vi "Init.vi"(8 "error in (no error)":errorcluster, 11 "reference in":refnum<class "Switch_Manager.lvclass">) -> (0 "error out":errorcluster, 3 "reference out":refnum<class "Switch_Manager.lvclass">)   [LabVIEW 2022 SP3, in "Switch_Manager.lvlib" / "Switch_Manager.lvclass"]
uses:
  Switch_Manager.lvclass
  Components/SwitchBase.lvlibp/SwitchBase.lvclass
  protected/SwitchMap.ctl
  <userlib>/_OpenG.lib/array/array.llb/Search 1D Array (String)__ogtk.vi
  <userlib>/_OpenG.lib/array/array.llb/Delete Elements from 1D Array (String)__ogtk.vi
  <userlib>/_OpenG.lib/array/array.llb/Remove Duplicates from 1D Array (String)__ogtk.vi
  <userlib>/_OpenG.lib/array/array.llb/Delete Elements from 1D Array (Boolean)__ogtk.vi
  Components/ViPER.lvlibp/ViPER.lvclass
  C:/Projects/Medulla/ViPER/Examples/Flux_Capacitor_Tester/Components/ViPER.lvlibp/ViPER.lvclass
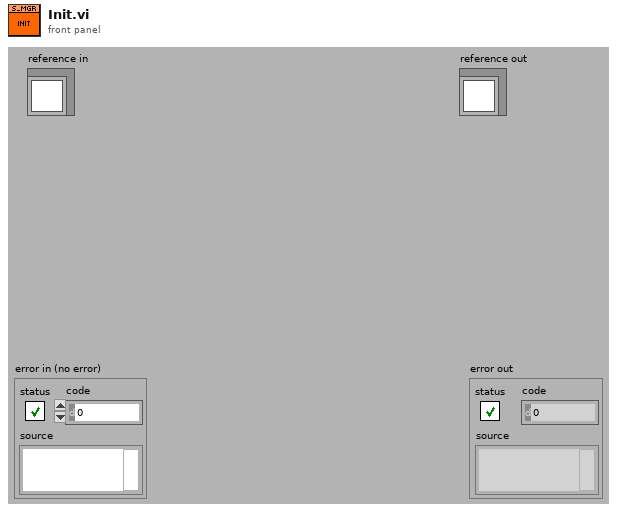
[diagram p1: front panel]
types:
  T1 = typedef "Switch_Manager.lvlib/Switch_Manager.lvclass/SwitchMap.ctl" = cluster{"Name":string, "Description":string, "Group":string, "IsGroup":bool, "Switches":string[]}
  T2 = cluster{"Ancestor":string, "Objects":refnum<class "ViPER.lvclass">[], "Object_Names":string[], "Owned":bool[]}[]
  T3 = cluster{"Ancestor":string, "Objects":refnum<class "ViPER.lvclass">[], "Object_Names":string[], "Owned":bool[]}
  T4 = cluster{"Name":string, "Description":string, "Group":string, "IsGroup":bool}[]
  T5 = typedef "Switch_Manager.lvlib/Switch_Manager.lvclass/ObjectAttributes.ctl" = cluster{"Config":T6, "State":bool[], "Switches":refnum<class "SwitchBase.lvclass">[], "SwitchName":string[], "SwitchMap":T1[], "UpdateEvent":refnum<user-event>, "ParentEvent":refnum<user-event>, "Tree":bool[]}
  T6 = typedef "Switch_Manager.lvlib/Switch_Manager.lvclass/Config.ctl" = cluster{"default":string}
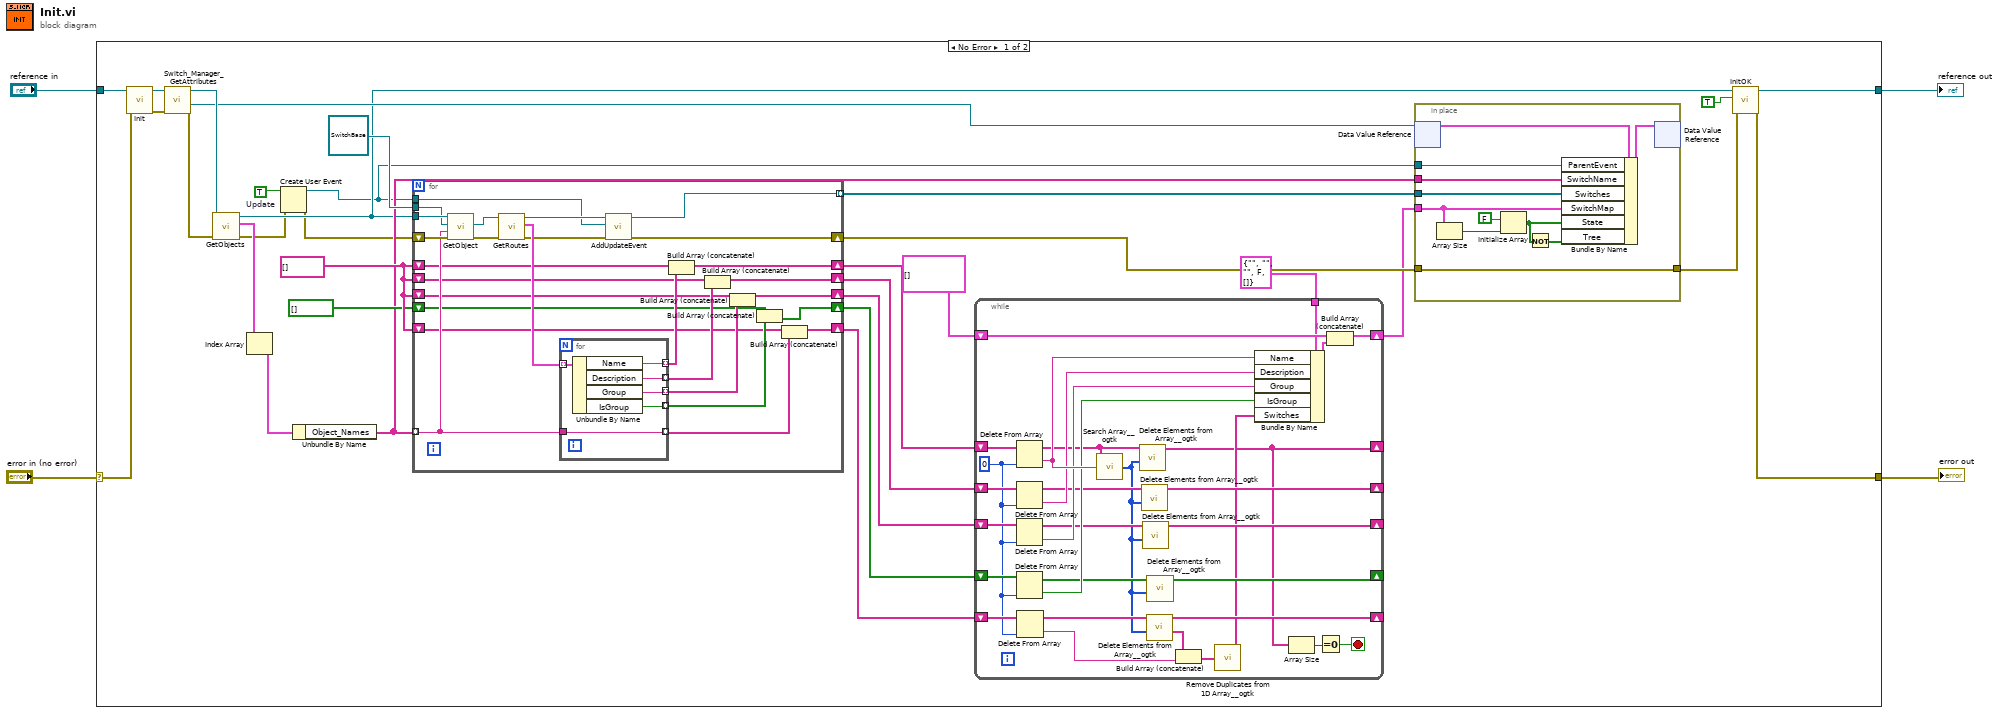
[diagram p0: block diagram]
diagram:
  n1 = case shown="No Error" "error in (no error)" {
    selector: "error in (no error)" -> [w35 w113]
    tunnel: [w30 w113] -> w3
    tunnel: [w32 w112] -> w1
    tunnel: "reference in" -> [w36 w112]
    frame No Error {
      w6 = TRUE  # Update
      w21 = string[] []
      n2 = call-parent "Init.vi"("error in (no error)"=w35, "reference in"=w36) -> ("error out"=w33:errorcluster, "reference out"=w34:refnum<class "Switch_Manager.lvclass">)  [unwired: 8 in]
      n3 = call "Switch_Manager_GetAttributes.vi"("error in (no error)"=w33, "reference in"=w34) -> ("error out"=w29:errorcluster, "DataRef"=w24:refnum<data-value>, "reference out"=w28:refnum<class "Switch_Manager.lvclass">)  [unwired: 6 in, 1 out]
      n4 = call "GetObjects.vi"("error in (no error)"=w29, "reference in"=w28) -> ("error out"=w8:errorcluster, "Ancestors"=w26:T2, "reference out"=w10:refnum<class "Switch_Manager.lvclass">)  [unwired: 7 in]
      n5 = Index Array(array=w26) -> (element=w25:T3)  [unwired: 1 in]
      n6 = Create User Event(user event datatype=w6, error in=w8) -> (user event=w5:refnum<user-event>, error out=w7:errorcluster)
      n7 = Unbundle By Name(w25) -> ("Object_Names"=w12:string[])
      n8 = for {
        tunnel: w10 -> [w94]
        tunnel: refnum<class "SwitchBase.lvclass"> refnum ("SwitchBase.lvlibp:reference") -> [w92]
        tunnel: w12 -> [w88] mode=indexing
        shift-right: [w71] -> w23
        shift-left: w7 -> [w93]
        tunnel: [w69] -> w22 mode=indexing
        shift-right: [w85] -> w19
        shift-left: w21 -> [w87]
        shift-right: [w82] -> w16
        shift-left: w21 -> [w84]
        shift-right: [w79] -> w15
        shift-left: w21 -> [w81]
        shift-right: [w76] -> w14
        shift-left: bool[] [] -> [w78]
        shift-right: [w73] -> w13
        shift-left: w21 -> [w75]
        tunnel: w5 -> [w68]
        n9 = call "GetObject.vi"("error in (no error)"=w93, "Object Name"=w88, "Class type"=w92, "reference in"=w94) -> ("error out"=w91:errorcluster, "Object out"=w90:refnum<class "SwitchBase.lvclass">)  [unwired: 5 in, 1 out]
        n10 = call-dynamic "GetRoutes.vi"("error in (no error)"=w91, "reference in"=w90) -> ("error out"=w72:errorcluster, "Routes"=w89:T4, "reference in"=w70:refnum<class "SwitchBase.lvclass">)  [unwired: 7 in]
        n11 = for {
          tunnel: w89 -> [w100] mode=indexing
          tunnel: w88 -> [w95]
          tunnel: [w99] -> w86 mode=indexing
          tunnel: [w98] -> w83 mode=indexing
          tunnel: [w97] -> w80 mode=indexing
          tunnel: [w96] -> w77 mode=indexing
          tunnel: [w95] -> w74 mode=indexing
          n12 = Unbundle By Name(w100) -> ("Name"=w99:string, "Description"=w98:string, "Group"=w97:string, "IsGroup"=w96:bool)
        }
        n13 = call-dynamic "AddUpdateEvent.vi"("error in (no error)"=w72, "UpdateEvent"=w68, "reference in"=w70) -> ("error out"=w71:errorcluster, "reference in"=w69:refnum<class "SwitchBase.lvclass">)  [unwired: 7 in]
        n14 = Build Array (concatenate)(w87, w86) -> (w85:string[])
        n15 = Build Array (concatenate)(w84, w83) -> (w82:string[])
        n16 = Build Array (concatenate)(w81, w80) -> (w79:string[])
        n17 = Build Array (concatenate)(w78, w77) -> (w76:bool[])
        n18 = Build Array (concatenate)(w75, w74) -> (w73:string[])
      }
      n19 = while {
        shift-right: [w41] -> _
        shift-left: w19 -> [w67]
        shift-right: [w65] -> w11
        shift-left: T1[] [] -> [w66]
        tunnel: T1 {"Name"="", "Description"="", "Group"="", "IsGroup"=FALSE, "Switches"=[]} -> [w64]
        shift-right: [w52] -> _
        shift-left: w16 -> [w62]
        shift-right: [w51] -> _
        shift-left: w15 -> [w60]
        shift-right: [w49] -> _
        shift-left: w14 -> [w59]
        shift-right: [w46] -> _
        shift-left: w13 -> [w55]
        stop <- w39 stop-if-true
        w37 = 0 ("index")
        n20 = Delete From Array(array=w67, index=w37) -> (deleted portion=w63:string, array with subset deleted=w56:string[])  [unwired: 1 in]
        n21 = Delete From Array(array=w62, index=w37) -> (deleted portion=w61:string, array with subset deleted=w54:string[])  [unwired: 1 in]
        n22 = Delete From Array(array=w60, index=w37) -> (deleted portion=w58:string, array with subset deleted=w53:string[])  [unwired: 1 in]
        n23 = Delete From Array(array=w59, index=w37) -> (deleted portion=w57:bool, array with subset deleted=w50:bool[])  [unwired: 1 in]
        n24 = Delete From Array(array=w55, index=w37) -> (deleted portion=w45:string, array with subset deleted=w48:string[])  [unwired: 1 in]
        n25 = call-poly <userlib>:"Search Array__ogtk.vi"("Array"=w56, "Element Data"=w63) -> ("Indices of Elements"=w44:i32[])  [unwired: 7 in]
        n26 = call-poly <userlib>:"Delete Elements from Array__ogtk.vi"("indices"=w44, "array"=w56) -> ("array w/ subset deleted"=w41:string[])  [unwired: 8 in, 1 out]
        n27 = call-poly <userlib>:"Delete Elements from Array__ogtk.vi"("indices"=w44, "array"=w54) -> ("array w/ subset deleted"=w52:string[])  [unwired: 8 in, 1 out]
        n28 = call-poly <userlib>:"Delete Elements from Array__ogtk.vi"("indices"=w44, "array"=w53) -> ("array w/ subset deleted"=w51:string[])  [unwired: 8 in, 1 out]
        n29 = call-poly <userlib>:"Delete Elements from Array__ogtk.vi"("indices"=w44, "array"=w48) -> ("deleted elements"=w47:string[], "array w/ subset deleted"=w46:string[])  [unwired: 8 in]
        n30 = call-poly <userlib>:"Delete Elements from Array__ogtk.vi"("indices"=w44, "array"=w50) -> ("array w/ subset deleted"=w49:bool[])  [unwired: 8 in, 1 out]
        n31 = Build Array (concatenate)(w47, w45) -> (w43:string[])
        n32 = call-poly <userlib>:"Remove Duplicates from 1D Array__ogtk.vi"("Input Array"=w43) -> ("Output Array"=w42:string[])  [unwired: 1 out]
        n33 = Bundle By Name(cluster=w64, "Name"=w63, "Description"=w61, "Group"=w58, "IsGroup"=w57, "Switches"=w42) -> (w38:T1)
        n34 = Array Size(array=w41) -> (size(s)=w40:i32)
        n35 = Equal To 0?(x=w40) -> (x = 0?=w39:bool)
        n36 = Build Array (concatenate)(w66, w38) -> (w65:T1[])
      }
      n37 = in-place {
        in-place-border: w23 -> [w107]
        in-place-border: w22 -> [w109]
        in-place-border: w12 -> [w108]
        in-place-border: w11 -> [w106]
        in-place-border: [w107] -> w9
        in-place-border: w5 -> [w103]
        n38 = in-place-dvr #1(w24) -> (w111:T5)  [unwired: 1 out]
        n39 = Array Size(array=w106) -> (size(s)=w104:i32)
        n40 = Initialize Array(FALSE, w104) -> (w102:bool[])
        n41 = Not(x=w102) -> (.not. x?=w101:bool[])
        n42 = Bundle By Name(cluster=w111, "ParentEvent"=w103, "SwitchName"=w108, "Switches"=w109, "SwitchMap"=w106, "State"=w102, "Tree"=w101) -> (w110:T5)
        n43 = in-place-dvr #1(w110) -> ()  [unwired: 2 out]
      }
      n44 = call "InitOK.vi"("error in (no error)"=w9, "Init OK?"=TRUE, "reference in"=w10) -> ("error out"=w30:errorcluster, "reference out"=w32:refnum<class "Switch_Manager.lvclass">)  [unwired: 7 in]
    }
    frame Error {
    }
  }
  "error out" <- w3
  "reference out" <- w1
